vi "Rundenzeit.vi"(11 "8 IR true":bool) -> (3 "output array":dbl[](array[numeric]))   [LabVIEW 2016]
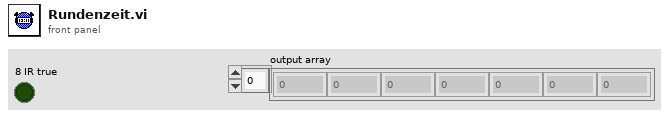
[diagram p1: front panel]
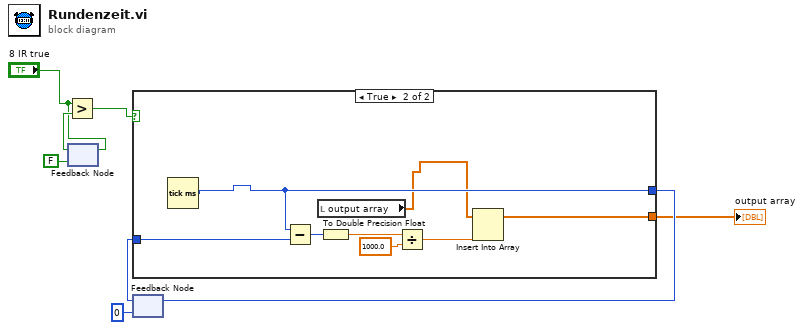
[diagram p0: block diagram]
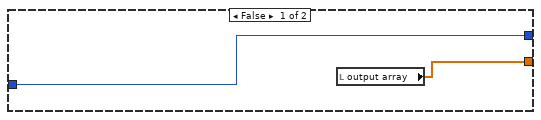
[diagram p2: hidden frame]
diagram:
  n1 = feedback #1(FALSE ("8 IR true")) -> (w5:bool)
  n2 = Greater?(x="8 IR true", y=w5) -> (0:w3:bool)
  n3 = feedback-in #1("8 IR true") -> ()
  n4 = feedback #2(u32 0 ("millisecond timer value")) -> (w7:u32)
  n5 = case shown="True" w3 {
    tunnel: [w10 w14] -> w8
    tunnel: w7 -> [w10 w18]
    tunnel: [w9 w12] -> w1
    frame False {
      n6 = local read "output array"() -> (w9:dbl[])
    }
    frame True {
      n7 = Tick Count (ms)() -> (millisecond timer value=w14:u32)
      n8 = Subtract(x=w14, y=w18) -> (x-y=w15:u32)
      n9 = local read "output array"() -> (w11:dbl[])
      n10 = To Double Precision Float(number=w15) -> (double precision float=w17:dbl)
      n11 = Divide(x=w17, y=1000.0) -> (x/y=w13:dbl)
      n12 = Insert Into Array(array=w11, new element=w13) -> (w12:dbl[])  [unwired: 1 in]
    }
  }
  "output array" <- w1
  n13 = feedback-in #2(w8) -> ()
